vi "fgv_imgbuf_raw.vi"(7 "cmd":enum16{"create", "close", "write", "read"}(ring), 8 "error in":errorcluster, 11 "raw Image in":T1) -> (0 "error out":errorcluster caption="error our", 3 "Image":T1(plugin-control))   [LabVIEW 2019]
uses:
  <vilib>/vision/Image Controls.llb/IMAQ Image.ctl
panel:
  out "raw image out":T1
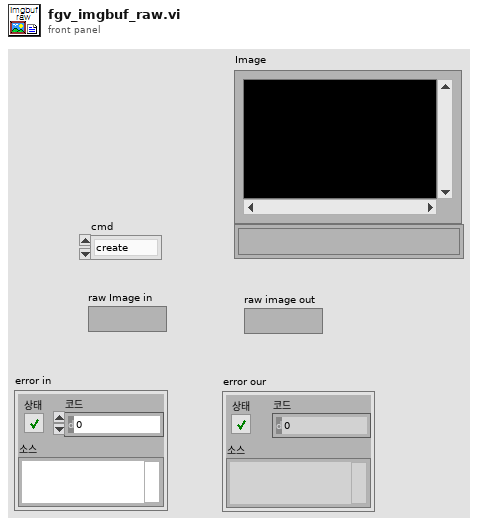
[diagram p1: front panel]
types:
  T1 = typedef "IMAQ Image.ctl" = refnum<image>
  T2 = typedef "Image Type" = u32
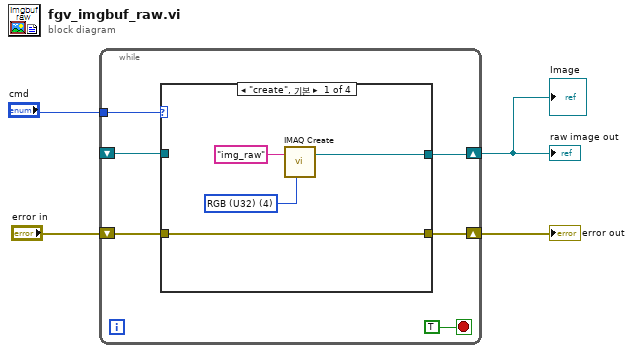
[diagram p0: block diagram]
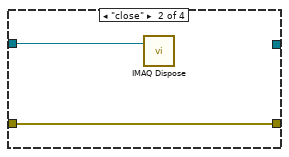
[diagram p2: hidden frame]
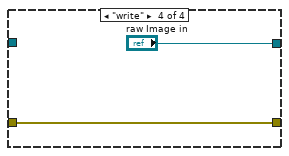
[diagram p4: hidden frame]
diagram:
  n1 = while {
    tunnel: "cmd" -> [w9]
    shift-right: [w8] -> w2
    shift-left: "error in" -> [w7]
    shift-right: [w6] -> w1
    shift-left: _ -> [w5]
    stop <- TRUE stop-if-true
    n2 = case shown="\"create\", 기본" w9 {
      tunnel: [w12 w16 w18 w20] -> w8
      tunnel: w7 -> [w12 w16 w18 w20]
      tunnel: [w13 _ w17 "raw Image in"] -> w6
      tunnel: w5 -> [_ w15 w17 _]
      frame "create", Default {
        w11 = T2 4 items=["Grayscale (U8)", "Grayscale (I16)", "Grayscale (SGL)", "Complex (CSG)", "RGB (U32)", "HSL (U32)", "RGB (U64)", "Grayscale (U16)"] ("Image Type")
        n3 = call "IMAQ Create"("Image Name"="img_raw", "Image Type"=w11) -> ("New Image"=w13:T1)  [unwired: 3 in, 1 out]
      }
      frame "close" {
        n4 = call "IMAQ Dispose"("Image"=w15) -> ()  [unwired: 5 in, 1 out]
      }
      frame "read" {
      }
      frame "write" {
      }
    }
  }
  "error out" <- w2
  "raw image out" <- w1
  "Image" <- w1
